vi "Read SMO Address.vi"(8 "error in (no error)":errorcluster, 11 "Instrument in":refnum<class "Instrument.lvclass">) -> (0 "error out":errorcluster, 1 "URI":string, 2 "Address":string, 3 "Instrument out":refnum<class "Instrument.lvclass">)   [LabVIEW 2019, in "Instrument.lvlib" / "Instrument.lvclass"]
uses:
  Instrument.lvclass
  Instrument.lvclass/Instrument.ctl
  <vilib>/JKI/JKI SMO/URI Parsing/URI.lvlib
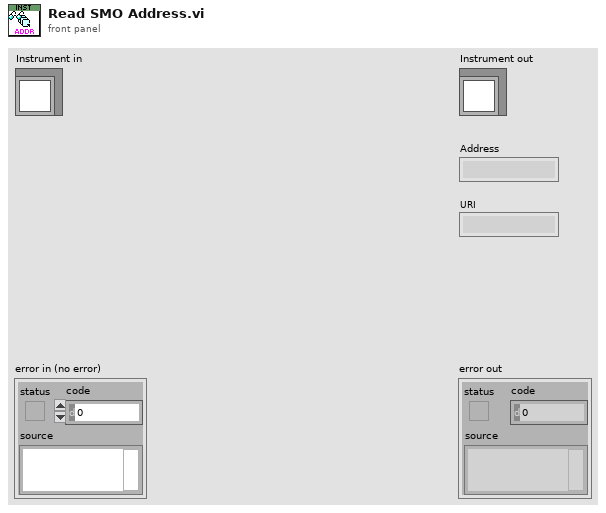
[diagram p1: front panel]
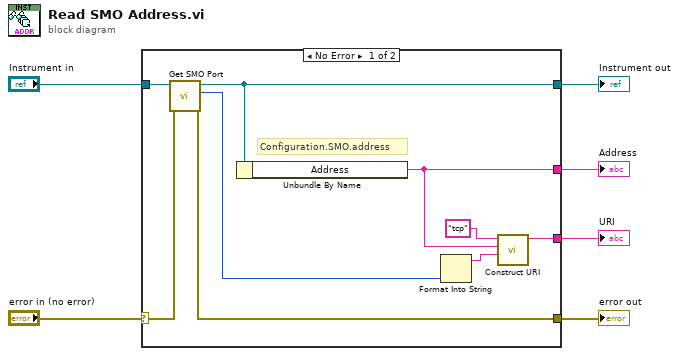
[diagram p0: block diagram]
diagram:
  n1 = case shown="No Error" "error in (no error)" {
    selector: "error in (no error)" -> [w11 w16]
    tunnel: [w10 w16] -> w5
    tunnel: [w9 w17] -> w3
    tunnel: "Instrument in" -> [w8 w17]
    tunnel: [w14 _] -> w2
    tunnel: [w12 _] -> w1
    frame No Error {
      # "Configuration.SMO.address"
      n2 = call-dynamic "Get SMO Port.vi"("error in (no error)"=w11, "Instrument in"=w8) -> ("error out"=w10:errorcluster, "Port"=w7:u16, "Instrument out"=w9:refnum<class "Instrument.lvclass">)  [unwired: 7 in]
      n3 = Unbundle By Name(w9) -> ("Address"=w14:string)
      n4 = Format Into String(w7) -> (resulting string=w13:string)  [unwired: 3 in, 1 out]
      n5 = call <vilib>:"Construct URI.vi"("port"=w13, "address"=w14, "protocol"="tcp") -> ("URI"=w12:string)  [unwired: 8 in]
    }
    frame Error {
    }
  }
  "error out" <- w5
  "Instrument out" <- w3
  "Address" <- w2
  "URI" <- w1
